vi "Read Message Flattener.vi"(11 "Message Stream in":refnum<class "Message Stream.lvclass">) -> (2 "Message Flattener.lvclass":refnum<class "Message Flattener.lvclass">, 3 "Message Stream out":refnum<class "Message Stream.lvclass">)   [LabVIEW 2020, in "Message Stream.lvclass"]
uses:
  Message Stream.lvclass
  Message Flattener/Message Flattener.lvclass
  Message Stream.lvclass/Message Stream.ctl
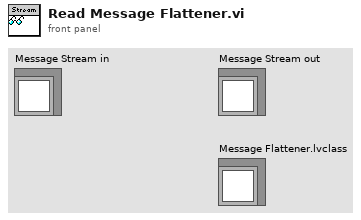
[diagram p1: front panel]
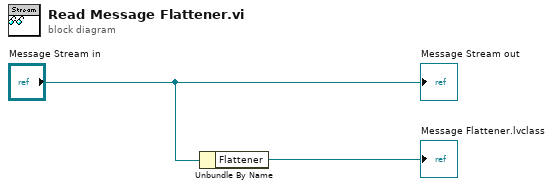
[diagram p0: block diagram]
diagram:
  n1 = Unbundle By Name("Message Stream in") -> ("Flattener"=→"Message Flattener.lvclass":refnum<class "Message Flattener.lvclass">)
  "Message Stream out" <- "Message Stream in"
